vi "Insert to Screen.vi"(8 "error in (no error)":errorcluster, 11 "Base UI Component in":refnum<class "Base UI Component.lvclass">) -> (0 "error out":errorcluster, 3 "Base UI Component out":refnum<class "Base UI Component.lvclass">)   [LabVIEW 2016, in "Assert Display.lvlib" / "Base UI Component.lvlib" / "Base UI Component.lvclass"]
uses:
  Base UI Component.lvclass
  Base UI Component.lvclass/Base UI Component.ctl
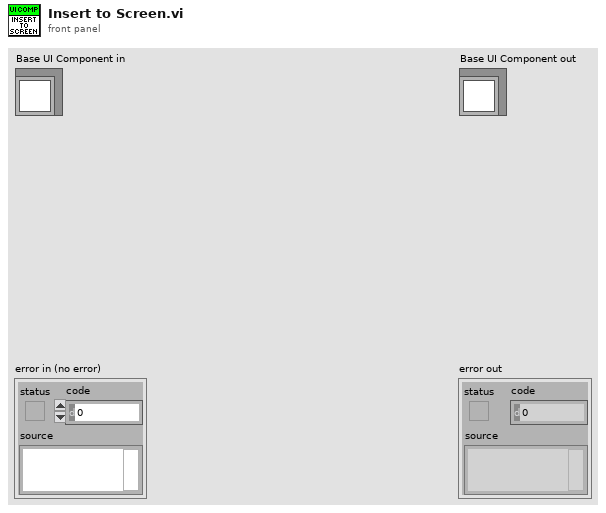
[diagram p1: front panel]
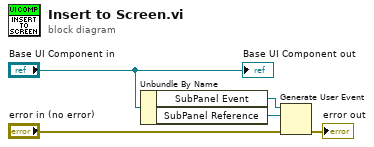
[diagram p0: block diagram]
diagram:
  n1 = Unbundle By Name("Base UI Component in") -> ("SubPanel Event"=w2:refnum<user-event>, "SubPanel Reference"=w1:refnum<vi>)
  n2 = Generate User Event(user event=w2, event data cluster=w1, error in="error in (no error)") -> (error out=→"error out":errorcluster)  [unwired: 1 in, 1 out]
  "Base UI Component out" <- "Base UI Component in"
